vi "LS-50 Stage Engine.vi"(0 "Unique Notifier Name":string="ASI", 11 "COM Port":string[](array[string])) -> ()   [LabVIEW 2016]
uses:
  Stages Controls/Stage Focus Control.ctl
  Stages Controls/Stage Status.ctl
  Stages Controls/Stage Notifier Element.ctl
  Stages Controls/Stage Actions.ctl
  <vilib>/Instr/_visa.llb/VISA Configure Serial Port (Instr).vi
panel:
  in  "Velocity 2":dbl=0.001
  in  "Abort":bool
  out "Position":dbl[](array[numeric])
  in  "Velocity":dbl(ring)=2.0 items=["SUPER SLOW"=0.0010000000474974513, "SLOW"=1.0, "MEDIUM"=2.0, "FAST"=3.0]
  out "Status":T1
  in  "Quit":bool
  in  "Focus Control":T2
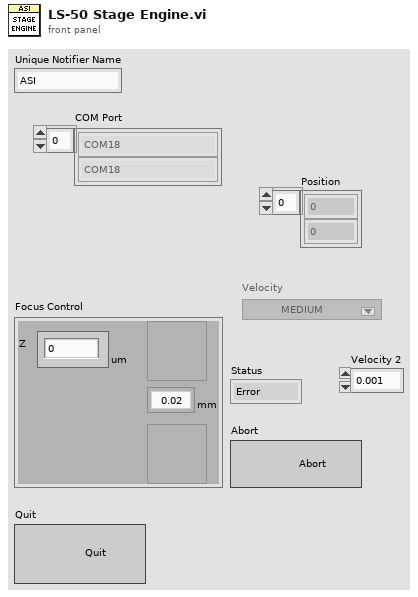
[diagram p1: front panel]
types:
  T1 = typedef "Stage Status.ctl" = enum16{"Error", "Abort", "Busy", "On Target"}
  T2 = typedef "Stage Focus Control.ctl" = cluster{"Focus Step (um)":enum16{"0.02", "0.05", "0.1", "0.5", "1", "2", "5", "10", "20"}, "Focus Up":bool, "Focus Down":bool, "Z ":dbl}
  T3 = typedef "Stage Actions.ctl" = enum16{"Get Position", "MVR", "MOVE", "HALT", "ONTARGET", "ERROR", "REFERENCE", "INIT", "VELOCITY", "STATUS", "EXIT", "HOME", "ZEROPOS", "NANOPOS", "ANALOG", "QUIT"}
  T4 = typedef "Stage Notifier Element.ctl" = cluster{"Action":T3, "Axis":bool[], "Setpoint":dbl[], "Velocity":dbl, "Cmd Recvd?":bool, "Position":dbl[], "Status":T1, "Misc":variant}
  T5 = cluster{"Focus Step (um)":bool, "Focus Up":bool, "Focus Down":bool, "Z ":bool}
  T6 = enum16{"0.02", "0.05", "0.1", "0.5", "1", "2", "5", "10", "20"}
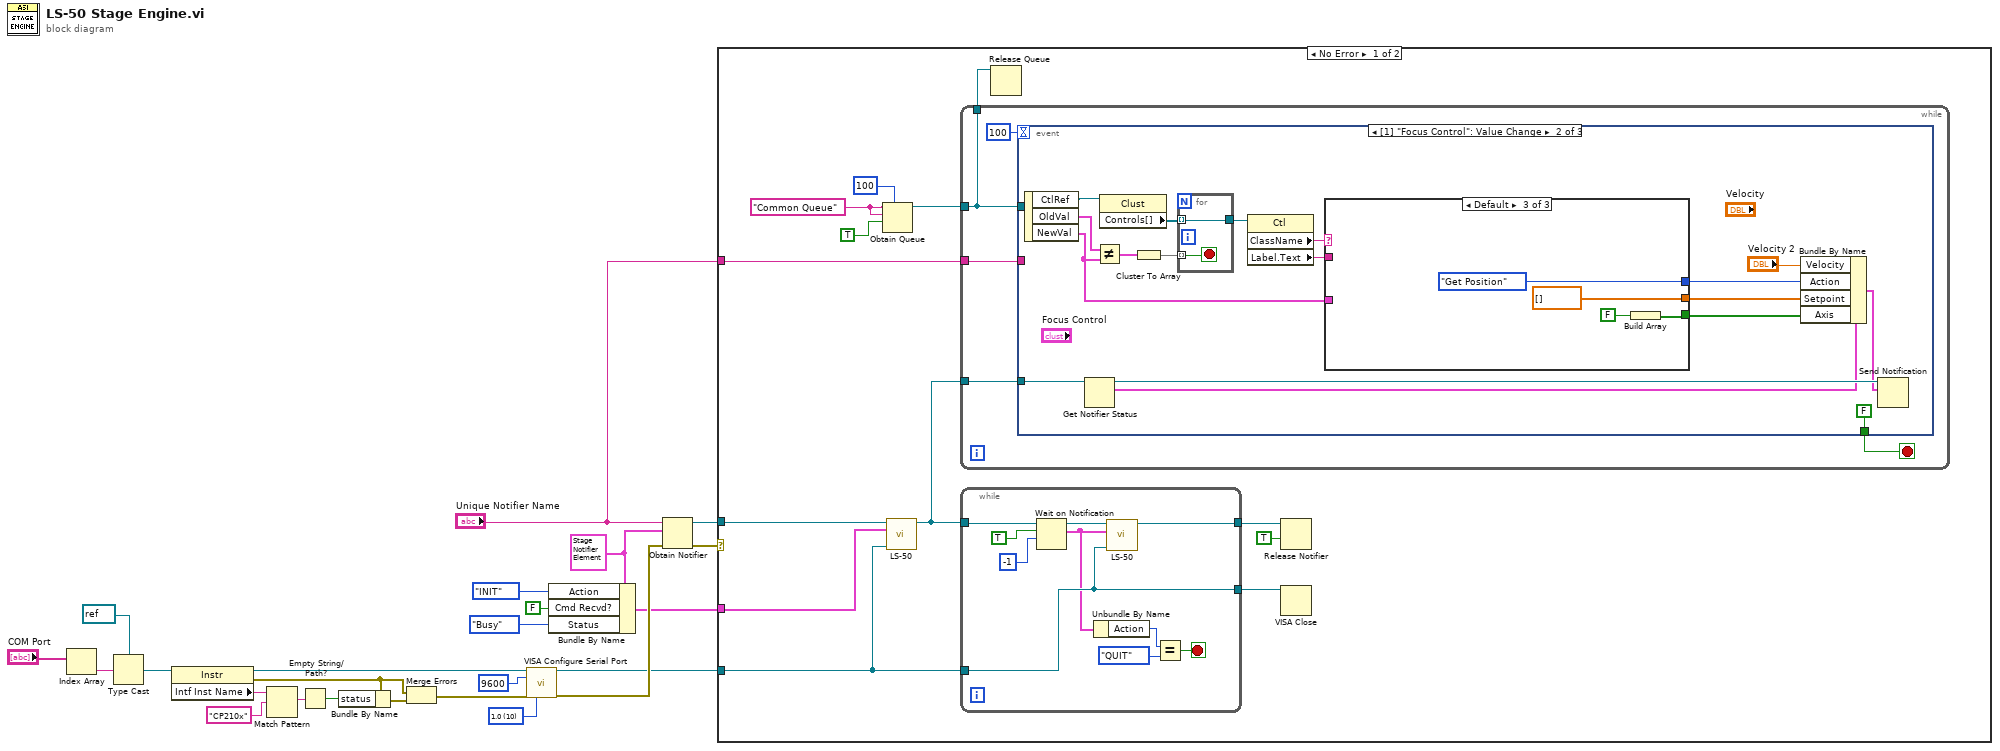
[diagram p0: block diagram]
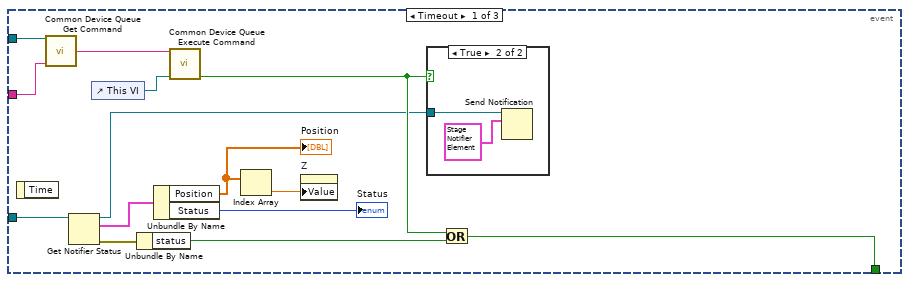
[diagram p2: hidden frame]
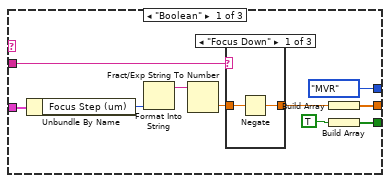
[diagram p4: hidden frame]
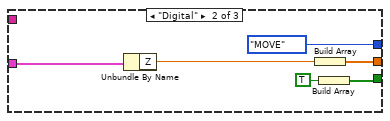
[diagram p7: hidden frame]
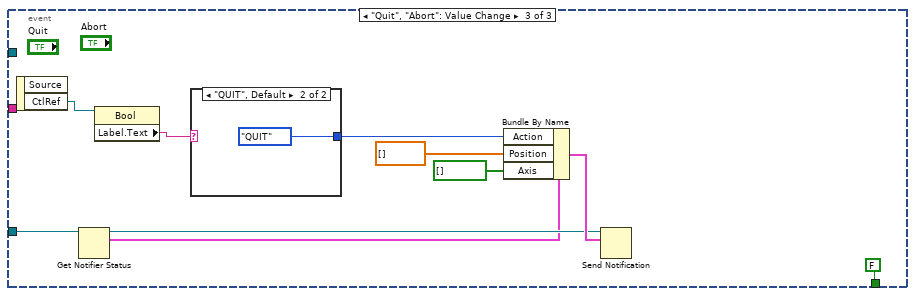
[diagram p8: hidden frame]
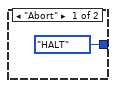
[diagram p9: hidden frame]
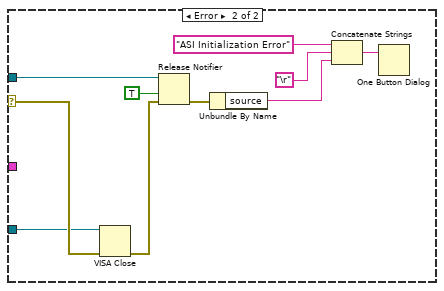
[diagram p10: hidden frame]
diagram:
  w10 = T4 {"Action"=enum."Get Position", "Axis"=[], "Setpoint"=[], "Velocity"=0.5, "Cmd Recvd?"=FALSE, "Position"=[], "Status"=enum."Abort", "Misc"=variant} ("Stage Status")
  w14 = u16 10 items=["1.0"=10, "1.5"=15, "2.0"=20] ("stop bits (10: 1 bit)")
  n1 = Index Array(array="COM Port") -> (element=w17:string)  [unwired: 1 in]
  n2 = Type Cast(type=refnum<visa-resource-name> refnum ("reference out"), x=w17) -> (*(type *) &x=w15:refnum<visa-resource-name>)
  n3 = property class="Instr"(reference=w15) -> (reference out=w12:refnum<visa-resource-name>, error out=w23:errorcluster, "Intf Inst Name"=w21:string)  [unwired: 1 in]
  n4 = Match Pattern(string=w21, regular expression="CP210x") -> (match substring=w19:string)  [unwired: 1 in, 3 out]
  n5 = Empty String/Path?(string/path=w19) -> (empty?=w22:bool)
  n6 = Bundle By Name(cluster=w23, "status"=w22) -> (w24:errorcluster)
  n7 = Merge Errors(w23, w24) -> (w11:errorcluster)
  n8 = call-poly "VISA Configure Serial Port"("VISA resource name"=w12, "baud rate (9600)"=u32 9600, "error in (no error)"=w11, "stop bits (10: 1 bit)"=w14) -> ("VISA resource name out"=w5:refnum<visa-resource-name>, "error out"=w6:errorcluster)  [unwired: 10 in]
  n9 = Bundle By Name(cluster=w10, "Action"=Stage_Actions."INIT", "Cmd Recvd?"=FALSE, "Status"=Stage_Status."Busy") -> (w2:T4)
  n10 = Obtain Notifier(name (unnamed)="Unique Notifier Name", notification data type=w10, error in (no error)=w6) -> (notifier out=w4:refnum<notifier>, error out=w3:errorcluster)  [unwired: 1 in, 1 out]
  n11 = case shown="No Error" w3 {
    selector: w3 -> [_ w126]
    tunnel: w5 -> [w29 w125]
    tunnel: w4 -> [w30 w127]
    tunnel: w2 -> [w25 _]
    tunnel: "Unique Notifier Name" -> [w27 _]
    frame No Error {
      w33 = "Common Queue" ("Unique Notifier Name")
      n12 = Obtain Queue(max queue size (-1, unlimited)=100, name (unnamed)=w33, element data type=w33, create if not found? (T)=TRUE) -> (queue out=w32:refnum<queue>)  [unwired: 1 in, 2 out]
      n13 = call "LS-50.vi"("LS-50 Notifier"=w30, "LS-50 Action"=w25, "LS-50 VISA"=w29) -> ("LS-50 Notifier (Dup)"=w28:refnum<notifier>)  [unwired: 12 in]
      n14 = while {
        tunnel: w28 -> [w50]
        tunnel: w32 -> [w49]
        tunnel: [w49] -> w31
        tunnel: w27 -> [w48]
        stop <- w51 stop-if-true
        n15 = event shown="[1] \"Focus Control\": Value Change" {
          selector: _ -> [_ _ _]
          dyn-events: _ -> [_ _ _]
          timeout: 100 -> [_ _ _]
          tunnel: [w57 FALSE ("status") FALSE ("status")] -> w51
          tunnel: w50 -> [w65 w74 w118]
          tunnel: w49 -> [w59 _ _]
          tunnel: w48 -> [w56 _ _]
          event Timeout {
            n16 = event-data() -> ()  [unwired: 1 in, 1 out]
            n17 = call "Common Device Queue Get Command.vi"("Common Queue"=w59, "Notifier Name"=w56) -> ("Command"=w60:string)  [unwired: 12 in, 1 out]
            n18 = Get Notifier Status(notifier=w65) -> (notifier out=w54:refnum<notifier>, current notification=w53:T4, error out=w63:errorcluster)  [unwired: 1 in, 2 out]
            n19 = control-ref of="This VI"() -> (w61:refnum<vi>)
            n20 = Unbundle By Name(w63) -> ("status"=w58:bool)
            n21 = Unbundle By Name(w53) -> ("Position"=w64:dbl[], "Status"=→"Status":T1)
            "Position" <- w64
            n22 = call "Common Device Queue Execute Command.vi"("Common Command"=w60, "VI Refnum"=w61) -> ("Quit?"=w55:bool)  [unwired: 12 in, 1 out]
            n23 = Index Array(array=w64) -> (element=w66:dbl)  [unwired: 1 in]
            n24 = property on="Z" class="DigNum (strict)"("Value"=w66) -> ()  [unwired: 2 in, 2 out]
            n25 = case shown="True" w55 {
              tunnel: w54 -> [_ w68]
              frame False {
              }
              frame True {
                n26 = Send Notification(notification=T4 {"Action"=enum."QUIT", "Axis"=[], "Setpoint"=[], "Velocity"=0.5, "Cmd Recvd?"=FALSE, "Position"=[], "Status"=enum."Error", "Misc"=variant} ("Stage Status"), notifier=w68) -> ()  [unwired: 1 in, 2 out]
              }
            }
            n27 = Or(x=w55, y=w58) -> (x .or. y?=w57:bool)
          }
          event Value Change {
            n28 = event-data() -> ("CtlRef"=w85:refnum<vi>, "OldVal"=w86:T2, "NewVal"=w79:T2)  [unwired: 1 in]
            n29 = Get Notifier Status(notifier=w74) -> (notifier out=w72:refnum<notifier>, current notification=w71:T4)  [unwired: 1 in, 3 out]
            n30 = Not Equal?(x=w86, y=w79) -> (x != y?=w84:T5)
            n31 = property class="Clust"(reference=w85) -> ("Controls[]"=w82:refnum<vi>[])  [unwired: 1 in, 2 out]
            n32 = Cluster To Array(cluster=w84) -> (array=w83:bool[])
            n33 = for {
              tunnel: w83 -> [w112] mode=indexing
              tunnel: [w111] -> w81
              tunnel: w82 -> [w111] mode=indexing
              stop <- w112 stop-if-true
            }
            n34 = property class="Ctl"(reference=w81) -> ("ClassName"=w80:string, "Label.Text"=w78:string)  [unwired: 1 in, 2 out]
            n35 = case shown="Default" w80 {
              tunnel: w79 -> [w94 w106 _]
              tunnel: w78 -> [w95 _ _]
              tunnel: [w89 w104 dbl[] []] -> w77
              tunnel: [w88 w103 w109] -> w76
              tunnel: [Stage_Actions."MVR" ("Action") Stage_Actions."MOVE" ("Action") Stage_Actions."Get Position" ("Action")] -> w73
              frame "Boolean" {
                n36 = Unbundle By Name(w94) -> ("Focus Step (um)"=w92:T6)
                n37 = Format Into String(w92) -> (resulting string=w93:string)  [unwired: 3 in, 1 out]
                n38 = Fract/Exp String To Number(string=w93) -> (number=w91:dbl)  [unwired: 3 in, 1 out]
                n39 = case shown="\"Focus Down\"" w95 {
                  tunnel: w91 -> [w98 w99 w100]
                  tunnel: [w97 w99 w100] -> w90
                  frame "Focus Down" {
                    n40 = Negate(x=w98) -> (-x=w97:dbl)
                  }
                  frame "Focus Up" {
                  }
                  frame Default {
                  }
                }
                n41 = Build Array(w90) -> (w89:dbl[])
                n42 = Build Array(TRUE) -> (w88:bool[])
              }
              frame "Digital" {
                n43 = Unbundle By Name(w106) -> ("Z"=w105:dbl)
                n44 = Build Array(w105) -> (w104:dbl[])
                n45 = Build Array(TRUE) -> (w103:bool[])
              }
              frame Default {
                n46 = Build Array(FALSE) -> (w109:bool[])
              }
            }
            n47 = Bundle By Name(cluster=w71, "Velocity"="Velocity 2", "Action"=w73, "Setpoint"=w77, "Axis"=w76) -> (w70:T4)
            n48 = Send Notification(notification=w70, notifier=w72) -> ()  [unwired: 1 in, 2 out]
          }
          event "Quit", "Abort": Value Change {
            n49 = event-data() -> ("CtlRef"=w114:refnum<vi>)  [unwired: 1 in, 1 out]
            n50 = Get Notifier Status(notifier=w118) -> (notifier out=w116:refnum<notifier>, current notification=w115:T4)  [unwired: 1 in, 3 out]
            n51 = property class="Bool"(reference=w114) -> ("Label.Text"=w113:string)  [unwired: 1 in, 2 out]
            n52 = case shown="\"QUIT\", Default" w113 {
              tunnel: [Stage_Actions."HALT" ("Action") Stage_Actions."QUIT" ("Action")] -> w117
              frame "Abort" {
              }
              frame "QUIT", Default {
              }
            }
            n53 = Bundle By Name(cluster=w115, "Action"=w117, "Position"=dbl[] [], "Axis"=bool[] []) -> (w119:T4)
            n54 = Send Notification(notification=w119, notifier=w116) -> ()  [unwired: 1 in, 2 out]
          }
        }
      }
      n55 = while {
        tunnel: w28 -> [w45]
        tunnel: [w40] -> w36
        tunnel: w29 -> [w39]
        tunnel: [w39] -> w26
        stop <- w47 stop-if-true
        n56 = Wait on Notification(notifier=w45, ignore previous (F)=TRUE, timeout in ms (-1)=-1) -> (notifier out=w41:refnum<notifier>, notification=w38:T4)  [unwired: 1 in, 2 out]
        n57 = Unbundle By Name(w38) -> ("Action"=w43:T3)
        n58 = call "LS-50.vi"("LS-50 Notifier"=w41, "LS-50 Action"=w38, "LS-50 VISA"=w39) -> ("LS-50 Notifier (Dup)"=w40:refnum<notifier>)  [unwired: 12 in]
        n59 = Equal?(x=w43, y=Stage_Actions."QUIT") -> (x = y?=w47:bool)
      }
      n60 = Release Queue(queue=w31) -> ()  [unwired: 2 in, 3 out]
      n61 = Release Notifier(notifier=w36, force destroy? (F)=TRUE) -> ()  [unwired: 1 in, 3 out]
      n62 = VISA Close(VISA resource name=w26) -> ()  [unwired: 1 in, 1 out]
    }
    frame Error {
      n63 = VISA Close(VISA resource name=w125, error in (no error)=w126) -> (error out=w128:errorcluster)
      n64 = Release Notifier(notifier=w127, force destroy? (F)=TRUE, error in (no error)=w128) -> (error out=w133:errorcluster)  [unwired: 2 out]
      n65 = Unbundle By Name(w133) -> ("source"=w130:string)
      n66 = Concatenate Strings("ASI Initialization Error", "\r", w130) -> (w129:string)
      n67 = One Button Dialog(message=w129) -> ()  [unwired: 1 in, 1 out]
    }
  }
